vi "Read BLRL Config.vi"(8 "error in (no error)":errorcluster, 11 "User BluelinesRedlines in":refnum<class "User BluelinesRedlines.lvclass">) -> (0 "error out":errorcluster, 2 "BLRL Config":T1, 3 "User BluelinesRedlines out":refnum<class "User BluelinesRedlines.lvclass">)   [LabVIEW 2020, in "VolatusGUIElements.lvlib" / "User BluelinesRedlines.lvclass"]
uses:
  User BluelinesRedlines.lvclass
  VolatusGUI/BluelinesRedlines Source/BLRL Config.ctl
  VolatusGUI/BluelinesRedlines Source/Range Limit Config.ctl
  User BluelinesRedlines.lvclass/User BluelinesRedlines.ctl
  VolatusGUI/BluelinesRedlines Source/BluelinesRedlines Source.lvclass
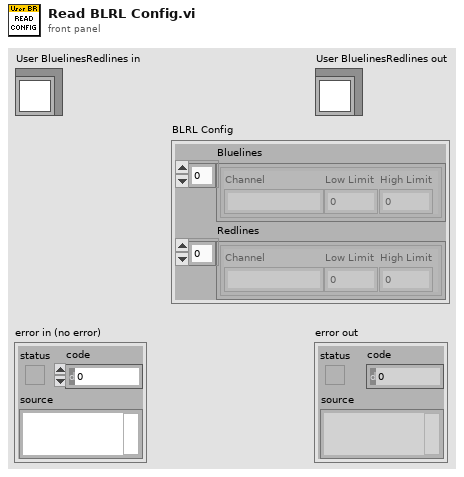
[diagram p1: front panel]
types:
  T1 = typedef "VolatusGUI.lvlib/BluelinesRedlines Source.lvclass/BLRL Config.ctl" = cluster{"Bluelines":T2[], "Redlines":T2[]}
  T2 = typedef "VolatusGUI.lvlib/BluelinesRedlines Source.lvclass/Range Limit Config.ctl" = cluster{"Channel":string, "Low Limit":dbl, "High Limit":dbl}
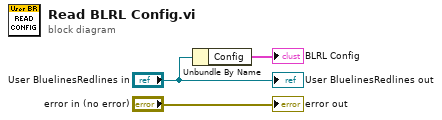
[diagram p0: block diagram]
diagram:
  n1 = Unbundle By Name("User BluelinesRedlines in") -> ("Config"=→"BLRL Config":T1)
  "error out" <- "error in (no error)"
  "User BluelinesRedlines out" <- "User BluelinesRedlines in"
